vi "setOnTheFlySpeed.vi"(0 "MultiAxisController in":refnum<class "_MultiAxisController.lvclass">, 2 "axis":T1, 3 "speed":i32, 5 "error in (no error)":errorcluster) -> (14 "MultiAxisController out":refnum<class "_MultiAxisController.lvclass">, 17 "success?":bool, 18 "response":string, 19 "error out":errorcluster)   [LabVIEW 2020, in "classes.lvlib" / "_MultiAxisController.lvclass"]
doc: "Produced By:\n\n<B>Kod Integrations, LLC</B>\n4835 Marianne Drive\nMount Airy, MD 21771\nhttp://www.kodintegrations.com\nemail: info@kodintegrations.com\nphone: (240) 687-1288"
uses:
  _MultiAxisController.lvclass
  C:/GEECS/Developers Version/source/Device Drivers/Newmark-NSC-A/Arcus Driver 3.0.0/ArcusUsbComm/classes/Controller/_Controller.lvclass
  axis.ctl
  _Controller.lvclass
  common.lvlib
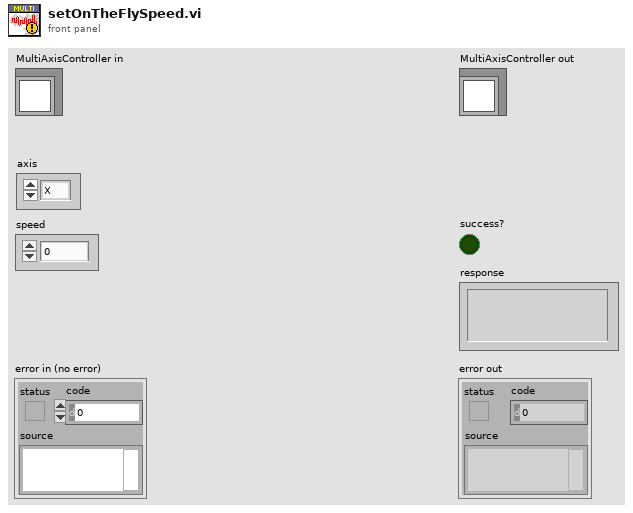
[diagram p1: front panel]
types:
  T1 = typedef "common.lvlib/axis.ctl" = enum16{"X", "Y", "Z", "U"}
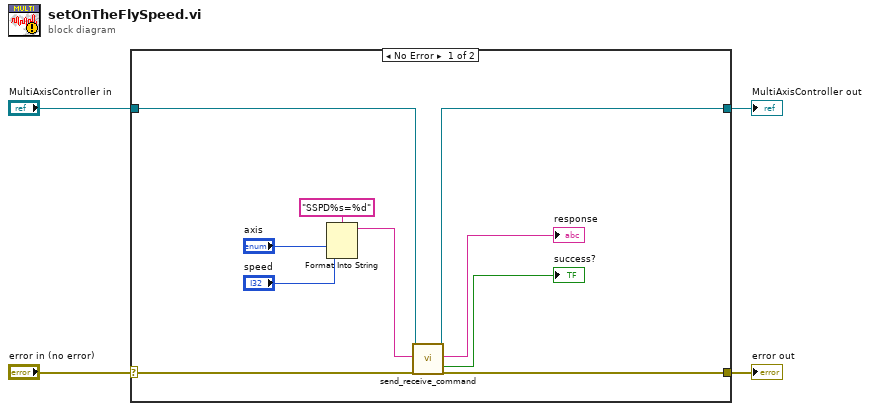
[diagram p0: block diagram]
diagram:
  n1 = case shown="No Error" "error in (no error)" {
    selector: "error in (no error)" -> [w9 w16]
    tunnel: [w8 w16] -> w3
    tunnel: [w6 w15] -> w1
    tunnel: "MultiAxisController in" -> [w7 w15]
    frame No Error {
      n2 = Format Into String(format string="SSPD%s=%d", "axis", "speed") -> (resulting string=w12:string)  [unwired: 2 in, 1 out]
      n3 = call "send_receive_command.vi"("reference (in)"=w7, "ASCII Command (in)"=w12, "error in (no error)"=w9) -> ("reference (out)"=w6:refnum<class "_MultiAxisController.lvclass">, "response (out)"=→"response":string, "success?"=→"success?":bool, "error out"=w8:errorcluster)  [unwired: 12 in, 1 out]
    }
    frame Error {
    }
  }
  "error out" <- w3
  "MultiAxisController out" <- w1
